vi "configrv.vi"(1 "rv":dbl, 2 "连接ID":refnum<k5>) -> (0 "连接ID输出":refnum<k5>)   [LabVIEW 2017]
panel:
  in  "输入簇":T1
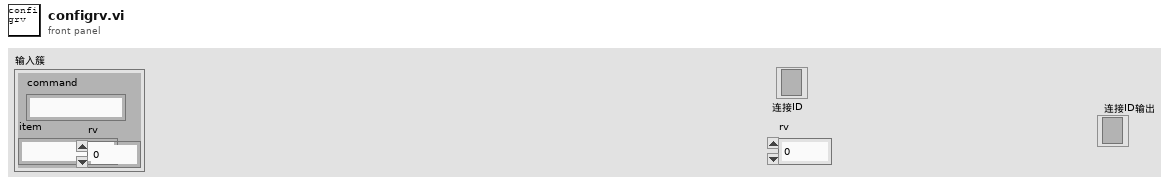
[diagram p1: front panel]
types:
  T1 = cluster{"command":string, "item":string, "rv":dbl}
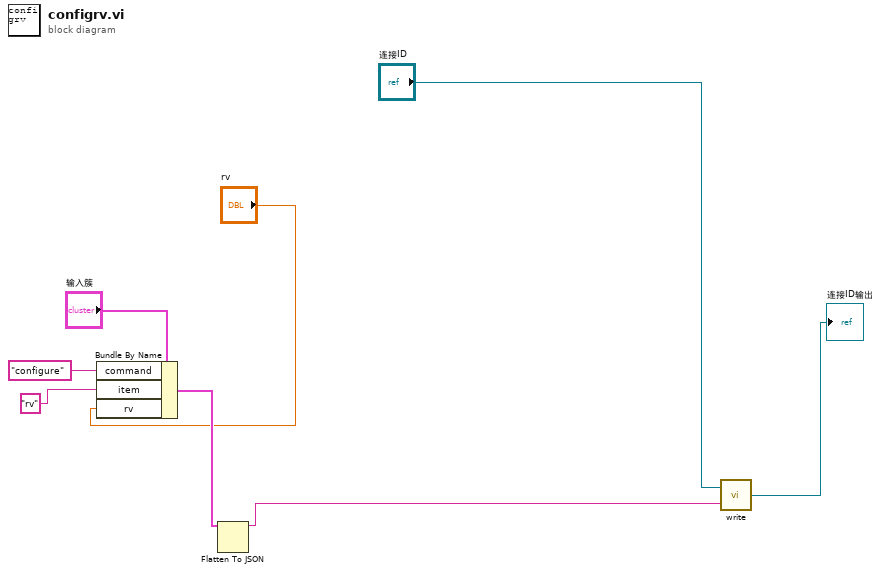
[diagram p0: block diagram]
diagram:
  n1 = Bundle By Name(cluster="输入簇", "command"="configure", "item"="rv" ("String"), "rv"="rv") -> (w3:T1)
  n2 = Flatten To JSON(anything=w3) -> (JSON string=w1:string)  [unwired: 2 in, 1 out]
  n3 = call "write.vi"("数据输入"=w1, "连接ID"="连接ID") -> ("连接ID输出"=→"连接ID输出":refnum<k5>)
